vi "Lock to LS.vi"(8 "error in (no error)":errorcluster, 10 "LockToLS":T1, 11 "Cfg Grandmaster in":refnum<class "Cfg Grandmaster.lvclass">) -> (0 "error out":errorcluster, 3 "Cfg Grandmaster out":refnum<class "Cfg Grandmaster.lvclass">)   [LabVIEW 2018, in "Configuration Grandmaster.lvlib" / "Cfg Grandmaster.lvclass"]
uses:
  Cfg Grandmaster.lvclass
  Common/Controls/LS Lock Sizes.ctl
  Cfg Grandmaster.lvclass/Cfg Grandmaster.ctl
  Class Chassis Cfg/ChassisCfg.lvclass
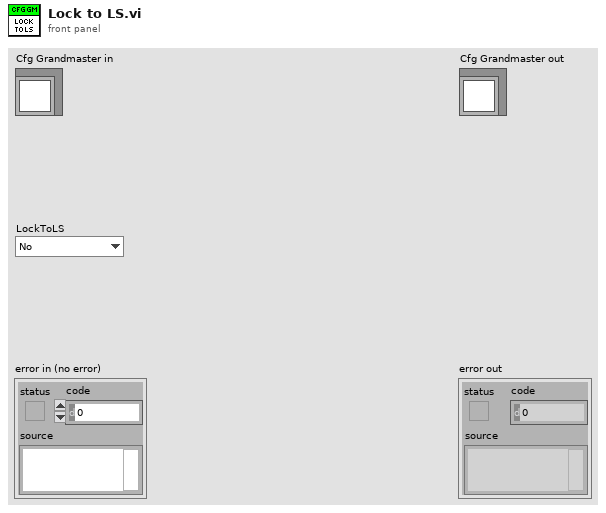
[diagram p1: front panel]
types:
  T1 = typedef "LS Lock Sizes.ctl" = enum16{"No", "250ms", "500ms", "1s"}
  T2 = typedef "ge_Cfg wChassis.ctl" = cluster{"Chassis BOM":refnum<class "Chassis BOM.lvclass">, "Chassis Cfg":refnum<class "ChassisCfg.lvclass">, "Chassis Tasks":refnum<class "Chassis Tasks.lvclass">, "HW Error":bool, "Unsvd Chgs?":bool}
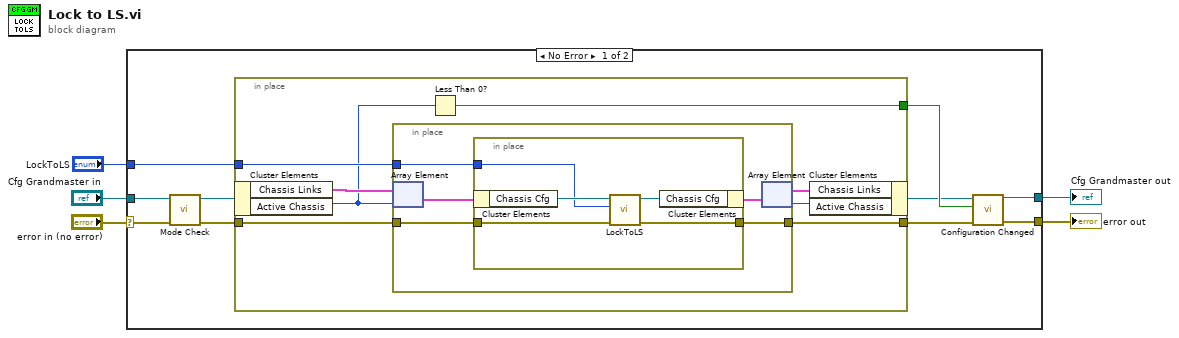
[diagram p0: block diagram]
diagram:
  n1 = case shown="No Error" "error in (no error)" {
    selector: "error in (no error)" -> [w11 w35]
    tunnel: [w9 w35] -> w4
    tunnel: [w8 w34] -> w2
    tunnel: "Cfg Grandmaster in" -> [w14 w34]
    tunnel: "LockToLS" -> [w15 _]
    frame No Error {
      n2 = call "Mode Check.vi"("error in (no error)"=w11, "Cfg Grandmaster in"=w14) -> ("error out"=w12:errorcluster, "Cfg Grandmaster out"=w13:refnum<class "Cfg Grandmaster.lvclass">)  [unwired: 8 in]
      n3 = in-place {
        in-place-border: w12 -> [w21]
        in-place-border: [w20] -> w6
        in-place-border: w15 -> [w19]
        in-place-border: [w17] -> w10
        n4 = in-place-cluster #1(w13) -> ("Chassis Links"=w23:T2[], "Active Chassis"=w18:i32)
        n5 = in-place {
          in-place-border: [w28] -> w20
          in-place-border: w21 -> [w27]
          in-place-border: w19 -> [w24]
          n6 = in-place-array #2(w23, w18) -> (w26:T2)
          n7 = in-place {
            in-place-border: w27 -> [w33]
            in-place-border: [w32] -> w28
            in-place-border: w24 -> [w29]
            n8 = in-place-cluster #3(w26) -> ("Chassis Cfg"=w31:refnum<class "ChassisCfg.lvclass">)
            n9 = call "LockToLS.vi"("error in (no error)"=w33, "LockToLS"=w29, "ChassisCfg"=w31) -> ("error out"=w32:errorcluster, "ChassisCfg"=w30:refnum<class "ChassisCfg.lvclass">)  [unwired: 7 in]
            n10 = in-place-cluster #3("Chassis Cfg"=w30) -> (w25:T2)
          }
          n11 = in-place-array #2(w25) -> (w22:T2[], w16:i32)
        }
        n12 = Less Than 0?(x=w18) -> (x < 0?=w17:bool)
        n13 = in-place-cluster #1("Chassis Links"=w22, "Active Chassis"=w16) -> (w7:refnum<class "Cfg Grandmaster.lvclass">)
      }
      n14 = call "Configuration Changed.vi"("error in (no error)"=w6, "Canceled? (F)"=w10, "Cfg Grandmaster in"=w7) -> ("error out"=w9:errorcluster, "Cfg Grandmaster out"=w8:refnum<class "Cfg Grandmaster.lvclass">)  [unwired: 7 in]
    }
    frame Error {
    }
  }
  "error out" <- w4
  "Cfg Grandmaster out" <- w2
